vi "PLC_Read_REAL_COLDEX.vi"(4 "address":i32, 6 "areaType":T1=132 items=["P Area"=128, "I Area"=129, "O Area"=130, "M Area"=131, "DB Area"=132, "Counter Area"=40, "Timer Area"=41], 7 "cpProtocol":i32=122, 8 "Error In":errorcluster, 9 "slot":i32=2, 10 "dataBlock":i32=31, 11 "ip":string="172.18.214.231") -> (0 "Error Out":errorcluster, 3 "Display":sgl)   [LabVIEW 2014]
uses:
  PLC_Libnodave_wrapper_areaType.ctl
panel:
  out "outBuffer":u8[](array[numeric])
  # "PLC Convert Data (1 REAL - 4 bytes)"
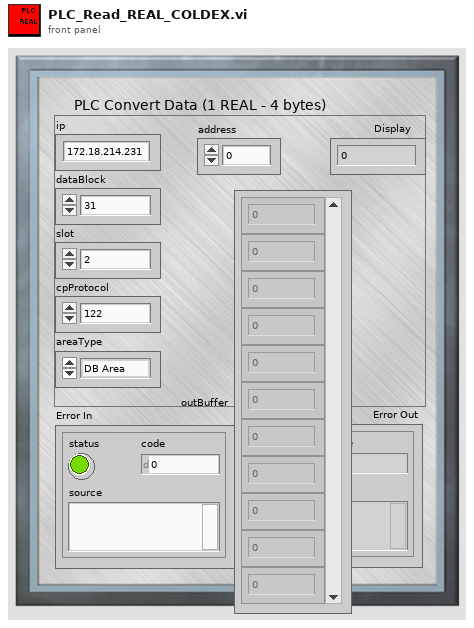
[diagram p1: front panel]
types:
  T1 = typedef "PLC_Libnodave_wrapper_areaType.ctl" = i32
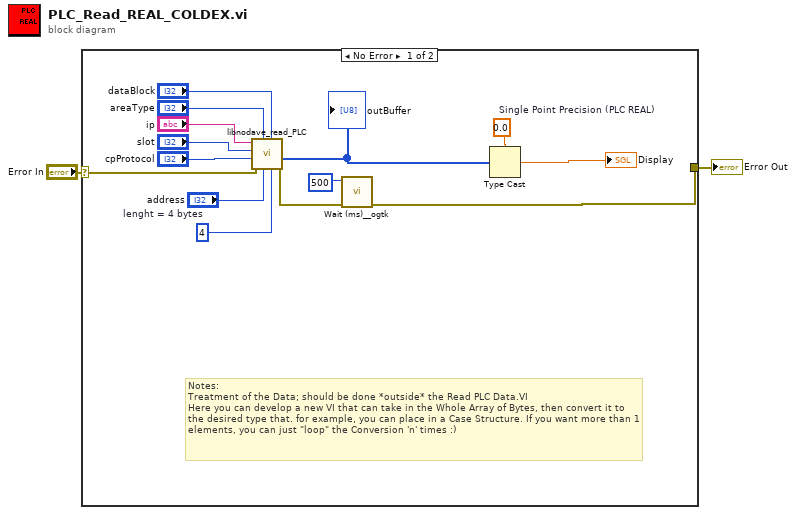
[diagram p0: block diagram]
diagram:
  n1 = case shown="No Error" "Error In" {
    selector: "Error In" -> [w16 w17]
    tunnel: [w6 w17] -> w1
    frame No Error {
      w8 = 4  # lenght = 4 bytes
      w10 = sgl 0.0  # Single Point Precision (PLC REAL)
      # "Notes:\nTreatment of the Data; should be done *outside* the Read PLC Data.VI\nHere you can develop a new VI that can take in the Whole Array of Bytes, then convert it to the desired type that. for example, you can place in a Case Structure. If you want more than 1 elements, you can just \"loop\" the Conversion 'n' times :)"
      n2 = call "libnodave_read_PLC.vi"("length"=w8, "dataBlock"="dataBlock", "start"="address", "areaType"="areaType", "Error In"=w16, "cpProtocol"="cpProtocol", "slot"="slot", "ip"="ip") -> ("Error Out"=w7:errorcluster, "outBuffer"=w4:u8[])  [unwired: 2 out]
      "outBuffer" <- w4
      n3 = call <userlib>:"Wait (ms)__ogtk.vi"("error in (no error)"=w7, "milliseconds to wait"=u32 500) -> ("error out"=w6:errorcluster)  [unwired: 8 in, 1 out]
      n4 = Type Cast(type=w10, x=w4) -> (*(type *) &x=→"Display":sgl)
    }
    frame Error {
    }
  }
  "Error Out" <- w1
